vi "Convert_ChannelReferenceArray_2_InstrumentReferenceArray.vi"(2 "error in":errorcluster, 3 "DCPowerInformation_byChannel_input":T2(array[cluster])) -> (0 "error out":errorcluster, 1 "DCPower_byInstrument_output":T1(array[cluster]))   [LabVIEW 2019]
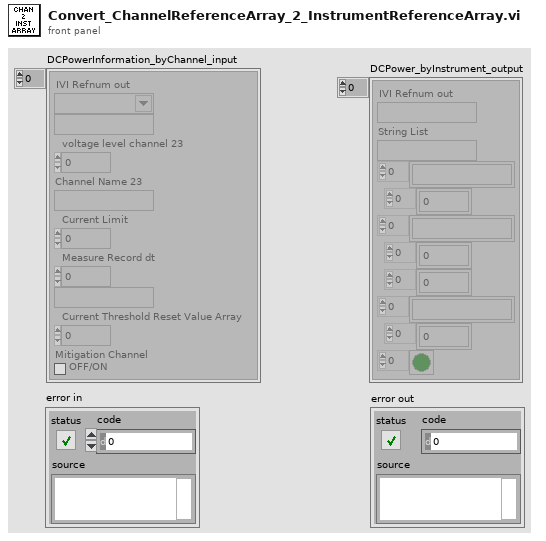
[diagram p1: front panel]
types:
  T1 = cluster{"IVI Refnum out":refnum<k15>, "String List":string, string[], dbl[], string[], dbl[], dbl[], string[], dbl[], bool[]}[]
  T2 = cluster{"IVI Refnum out":refnum<k15>, string, "voltage level channel 23":dbl, "Channel Name 23":string, "Current Limit":dbl, "Measure Record dt":dbl, string, "Current Threshold Reset Value Array":dbl, "Mitigation Channel":bool}[]
  T3 = cluster{"IVI Refnum out":refnum<k15>, string, "voltage level channel 23":dbl, "Channel Name 23":string, "Current Limit":dbl, "Measure Record dt":dbl, string, "Current Threshold Reset Value Array":dbl}[]
  T4 = cluster{"IVI Refnum out":refnum<k15>, string[], dbl[], string[], dbl[], dbl[], string[], dbl[], bool[]}[]
  T5 = cluster{"IVI Refnum out":refnum<k15>, string[], dbl[], string[], dbl[], dbl[], string[], dbl[], bool[]}
  T6 = cluster{"IVI Refnum out":refnum<k15>, "String List":string, string[], dbl[], string[], dbl[], dbl[], string[], dbl[], bool[]}
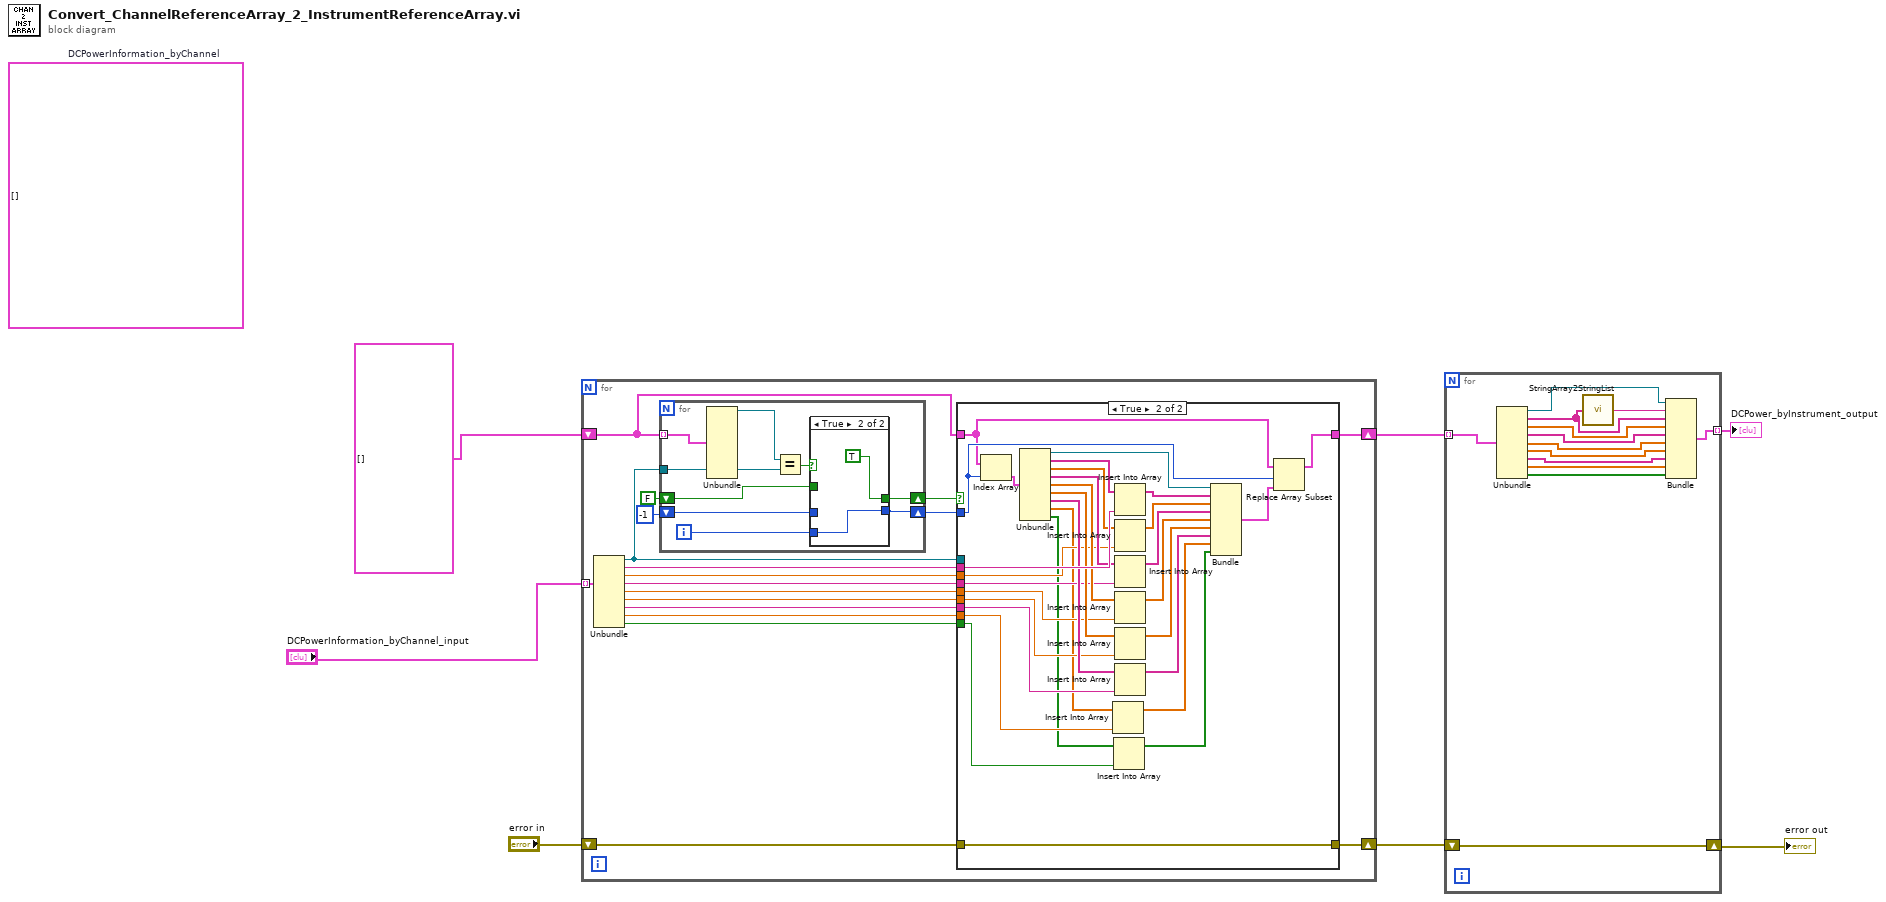
[diagram p0: block diagram]
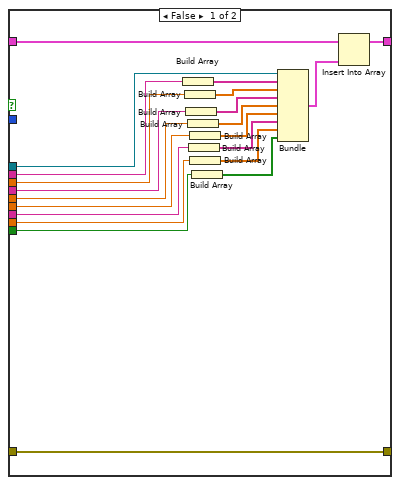
[diagram p3: hidden frame]
diagram:
  (unwired) T3 []  # DCPowerInformation_byChannel
  n1 = for {
    tunnel: "DCPowerInformation_byChannel_input" -> [w25] mode=indexing
    shift-right: [w18] -> w7
    shift-left: T4 [] -> [w13]
    shift-right: [w11] -> w5
    shift-left: "error in" -> [w10]
    n2 = Unbundle(w25) -> ("IVI Refnum out"=w17:refnum<k15>, w24:string, "voltage level channel 23"=w23:dbl, "Channel Name 23"=w22:string, "Current Limit"=w21:dbl, "Measure Record dt"=w20:dbl, w19:string, "Current Threshold Reset Value Array"=w9:dbl, "Mitigation Channel"=w8:bool)
    n3 = for {
      tunnel: w13 -> [w34] mode=indexing
      tunnel: w17 -> [w33]
      shift-right: [w30] -> w15
      shift-left: FALSE -> [w29]
      shift-right: [w28] -> w14
      shift-left: -1 -> [w26]
      i -> [w27]
      n4 = Unbundle(w34) -> ("IVI Refnum out"=w32:refnum<k15>)  [unwired: 8 out]
      n5 = Equal?(x=w32, y=w33) -> (x = y?=w31:bool)
      n6 = case shown="True" w31 {
        tunnel: [w36 TRUE] -> w30
        tunnel: w29 -> [w36 _]
        tunnel: [w35 w38] -> w28
        tunnel: w27 -> [_ w38]
        tunnel: w26 -> [w35 _]
        frame False {
        }
        frame True {
        }
      }
    }
    n7 = case shown="True" w15 {
      tunnel: w17 -> [w59 _]
      tunnel: w24 -> [w55 w88]
      tunnel: w23 -> [w52 w81]
      tunnel: w22 -> [w51 w80]
      tunnel: w21 -> [w49 w79]
      tunnel: w20 -> [w47 w78]
      tunnel: w19 -> [w45 w77]
      tunnel: [w57 w67] -> w18
      tunnel: w13 -> [w56 w74]
      tunnel: w14 -> [_ w75]
      tunnel: [w43 w66] -> w11
      tunnel: w10 -> [w43 w66]
      tunnel: w9 -> [w42 w64]
      tunnel: w8 -> [w40 w62]
      frame False {
        n8 = Build Array(w55) -> (w54:string[])
        n9 = Build Array(w52) -> (w53:dbl[])
        n10 = Build Array(w51) -> (w50:string[])
        n11 = Build Array(w49) -> (w48:dbl[])
        n12 = Build Array(w45) -> (w44:string[])
        n13 = Build Array(w47) -> (w46:dbl[])
        n14 = Build Array(w42) -> (w41:dbl[])
        n15 = Build Array(w40) -> (w39:bool[])
        n16 = Bundle("IVI Refnum out"=w59, w54, w53, w50, w48, w46, w44, w41, w39) -> (w58:T5)  [unwired: 1 in]
        n17 = Insert Into Array(array=w56, new element=w58) -> (w57:T4)  [unwired: 1 in]
      }
      frame True {
        n18 = Index Array(array=w74, index=w75) -> (element=w84:T5)
        n19 = Unbundle(w84) -> ("IVI Refnum out"=w90:refnum<k15>, w89:string[], w87:dbl[], w86:string[], w85:dbl[], w83:dbl[], w82:string[], w65:dbl[], w61:bool[])
        n20 = Insert Into Array(array=w65, new element=w64) -> (w63:dbl[])  [unwired: 1 in]
        n21 = Insert Into Array(array=w61, new element=w62) -> (w60:bool[])  [unwired: 1 in]
        n22 = Insert Into Array(array=w89, new element=w88) -> (w73:string[])  [unwired: 1 in]
        n23 = Insert Into Array(array=w87, new element=w81) -> (w72:dbl[])  [unwired: 1 in]
        n24 = Insert Into Array(array=w86, new element=w80) -> (w71:string[])  [unwired: 1 in]
        n25 = Insert Into Array(array=w85, new element=w79) -> (w70:dbl[])  [unwired: 1 in]
        n26 = Insert Into Array(array=w83, new element=w78) -> (w69:dbl[])  [unwired: 1 in]
        n27 = Insert Into Array(array=w82, new element=w77) -> (w68:string[])  [unwired: 1 in]
        n28 = Bundle("IVI Refnum out"=w90, w73, w72, w71, w70, w69, w68, w63, w60) -> (w76:T5)  [unwired: 1 in]
        n29 = Replace Array Subset(array=w74, new element=w76, index=w75) -> (w67:T4)
      }
    }
  }
  n30 = for {
    tunnel: w7 -> [w103] mode=indexing
    tunnel: [w94] -> w1 mode=indexing
    shift-right: [w93] -> w4
    shift-left: w5 -> [w93]
    n31 = Unbundle(w103) -> ("IVI Refnum out"=w102:refnum<k15>, w100:string[], w99:dbl[], w98:string[], w97:dbl[], w96:dbl[], w95:string[], w92:dbl[], w91:bool[])
    n32 = call "StringArray2StringList.vi"("String Array"=w100) -> ("String List"=w101:string)
    n33 = Bundle("IVI Refnum out"=w102, "String List"=w101, w100, w99, w98, w97, w96, w95, w92, w91) -> (w94:T6)  [unwired: 1 in]
  }
  "error out" <- w4
  "DCPower_byInstrument_output" <- w1
